vi "流动字幕显示.vi"() -> ()   [LabVIEW 2014]
panel:
  in  "停止按钮":bool
  in  "滚动方式":enum32{"左", "暂停", "右"}(radio)
  in  "滚动速度":u32=10
  out "?":bool[][](array[boolean])
  in  "字幕内容":string="加油好男儿"
  # "默认速度10"
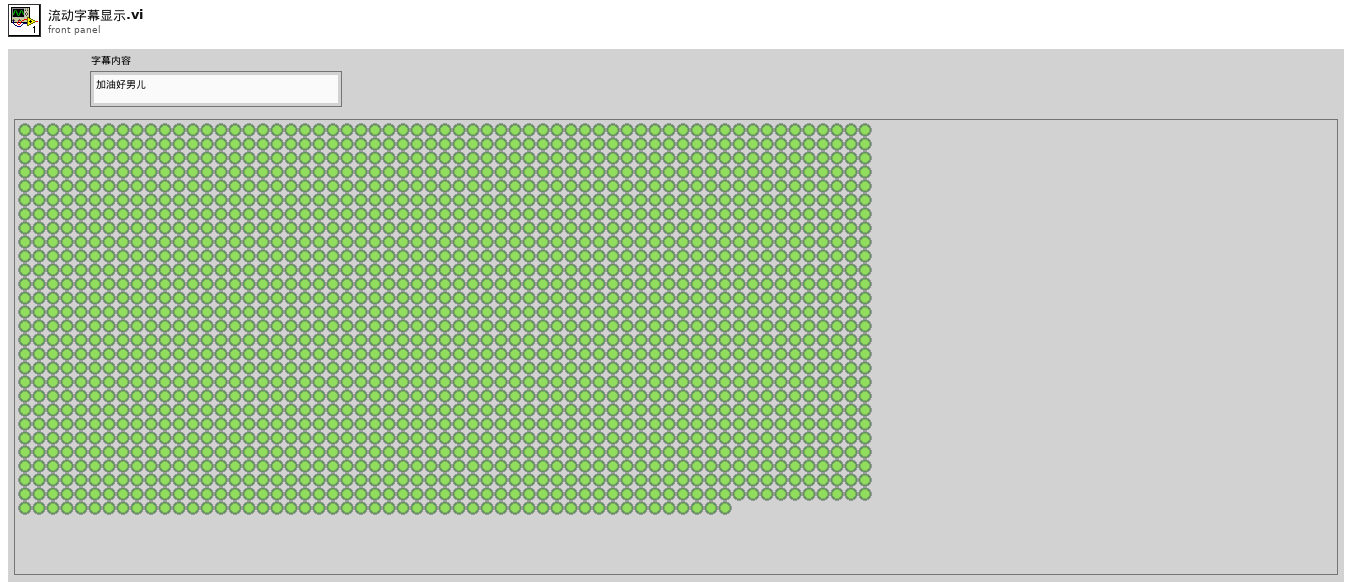
[diagram p1: front panel]
types:
  T1 = cluster{"left":i16, "top":i16, "right":i16, "bottom":i16}
  T2 = cluster{"Font Name:":string, "Size":i16, "Strikeout?":bool, "Italic?":bool, "Underline?":bool, "Outline?":bool, "Shadow?":bool, "Bold?":bool}
  T3 = enum16{"User-specified Font", "Application Font", "System Font", "Dialog Font"}
  T4 = typedef "imagedata.ctl" = cluster{"image type":i32, "image depth":i32, "image":u8[], "mask":u8[], "colors":u32[], "Rectangle":cluster{"left":i16, "top":i16, "right":i16, "bottom":i16}}
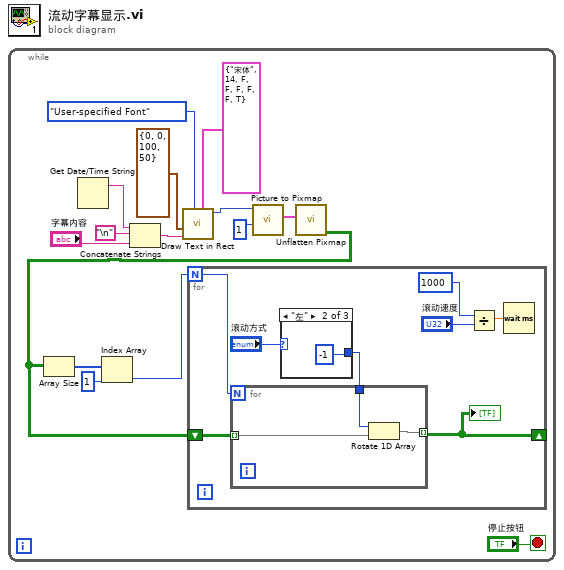
[diagram p0: block diagram]
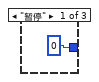
[diagram p2: hidden frame]
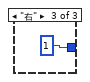
[diagram p3: hidden frame]
diagram:
  n1 = while {
    stop <- "停止按钮" stop-if-true
    n2 = Get Date/Time String() -> (date string=w2:string)  [unwired: 3 in, 1 out]
    n3 = Concatenate Strings(w2, "\n", "字幕内容") -> (w12:string)
    n4 = call <vilib>:"Draw Text in Rect.vi"("[user-specified font]"=T2 {"Font Name:"="宋体", "Size"=14, "Strikeout?"=FALSE, "Italic?"=FALSE, "Underline?"=FALSE, "Outline?"=FALSE, "Shadow?"=FALSE, "Bold?"=TRUE}, "desired font(Application)"=T3."User-specified Font", "text"=w12, "rect"=T1 {"left"=0, "top"=0, "right"=100, "bottom"=50}) -> ("new picture"=w15:picture)  [unwired: 7 in]
    n5 = call <vilib>:"Picture to Pixmap.vi"("depth"=1, "picture"=w15) -> ("image data"=w14:T4)  [unwired: 8 in, 1 out]
    n6 = call <vilib>:"Unflatten Pixmap.vi"("image data"=w14) -> ("1-bit pixmap"=w7:bool[][])  [unwired: 4 in, 6 out]
    n7 = Array Size(array=w7) -> (size(s)=w10:i32[])
    n8 = Index Array(array=w10, index=1 ("索引")) -> (element=w8:i32)
    n9 = for {
      N: w8 -> [w22]
      shift-right: [w21] -> _
      shift-left: w7 -> [w23]
      n10 = case shown="\"左\"" "滚动方式" {
        tunnel: [0 -1 1] -> w16
        frame "暂停" {
        }
        frame "左" {
        }
        frame "右" {
        }
      }
      n11 = for {
        N: w22 -> [_]
        tunnel: w23 -> [w29] mode=indexing
        tunnel: [w28] -> w21 mode=indexing
        tunnel: w16 -> [w27]
        n12 = Rotate 1D Array(1:w29, 2:w27) -> (0:w28:bool[])
      }
      "?" <- w21
      n13 = Divide(x=u32 1000 ("y"), y="滚动速度") -> (x/y=w20:dbl)
      n14 = Wait (ms)(milliseconds to wait=w20) -> ()  [unwired: 1 out]
    }
  }
